vi "Write Layout.vi"(8 "error in (no error)":errorcluster, 10 "Layout":T1={"Order"=enum."LeftRight", "Row"=2, "Column"=2, "Margin"=5}, 11 "ProjectBase in":refnum<class "Project.lvclass">) -> (0 "error out":errorcluster, 3 "ProjectBase out":refnum<class "Project.lvclass">)   [LabVIEW 2015, in "Project.lvclass"]
uses:
  Project.lvclass
  Project.lvclass/Project.ctl
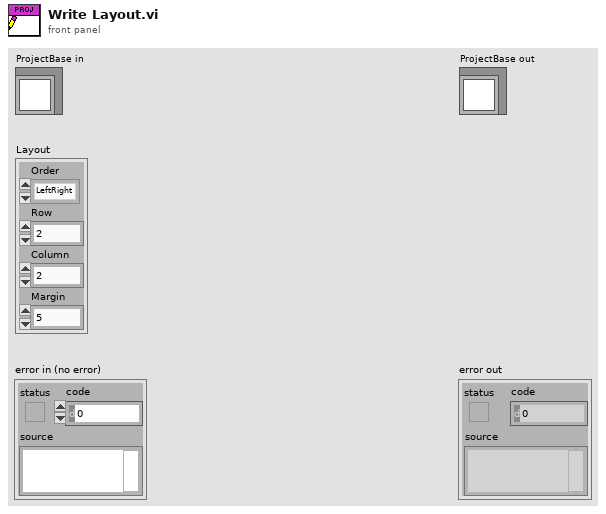
[diagram p1: front panel]
types:
  T1 = cluster{"Order":enum16{"LeftRight", "TopDown"}, "Row":i32, "Column":i32, "Margin":i32}
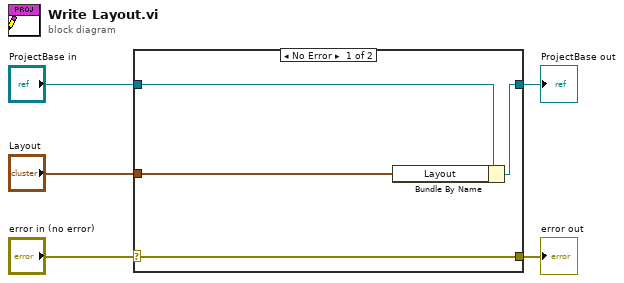
[diagram p0: block diagram]
diagram:
  n1 = case shown="No Error" "error in (no error)" {
    selector: "error in (no error)" -> [w9 w10]
    tunnel: [w9 w10] -> w4
    tunnel: [w7 w11] -> w2
    tunnel: "ProjectBase in" -> [w8 w11]
    tunnel: "Layout" -> [w6 _]
    frame No Error {
      n2 = Bundle By Name(cluster=w8, "Layout"=w6) -> (w7:refnum<class "Project.lvclass">)
    }
    frame Error {
    }
  }
  "error out" <- w4
  "ProjectBase out" <- w2
